vi "LoadOrCreateAParaIniCfg.vi"(8 "error in":errorcluster, 10 "Tree Refnum":refnum<vi>, 11 "Tbl Refnum in":refnum<vi>) -> (0 "error out":errorcluster, 1 "cfg file refnum out":refnum<file>, 2 "Tree Refnum out":refnum<vi>, 3 "Tbl Refnum out":refnum<vi>)   [LabVIEW 2010]
panel:
  out "All Tags":string[](array[string])
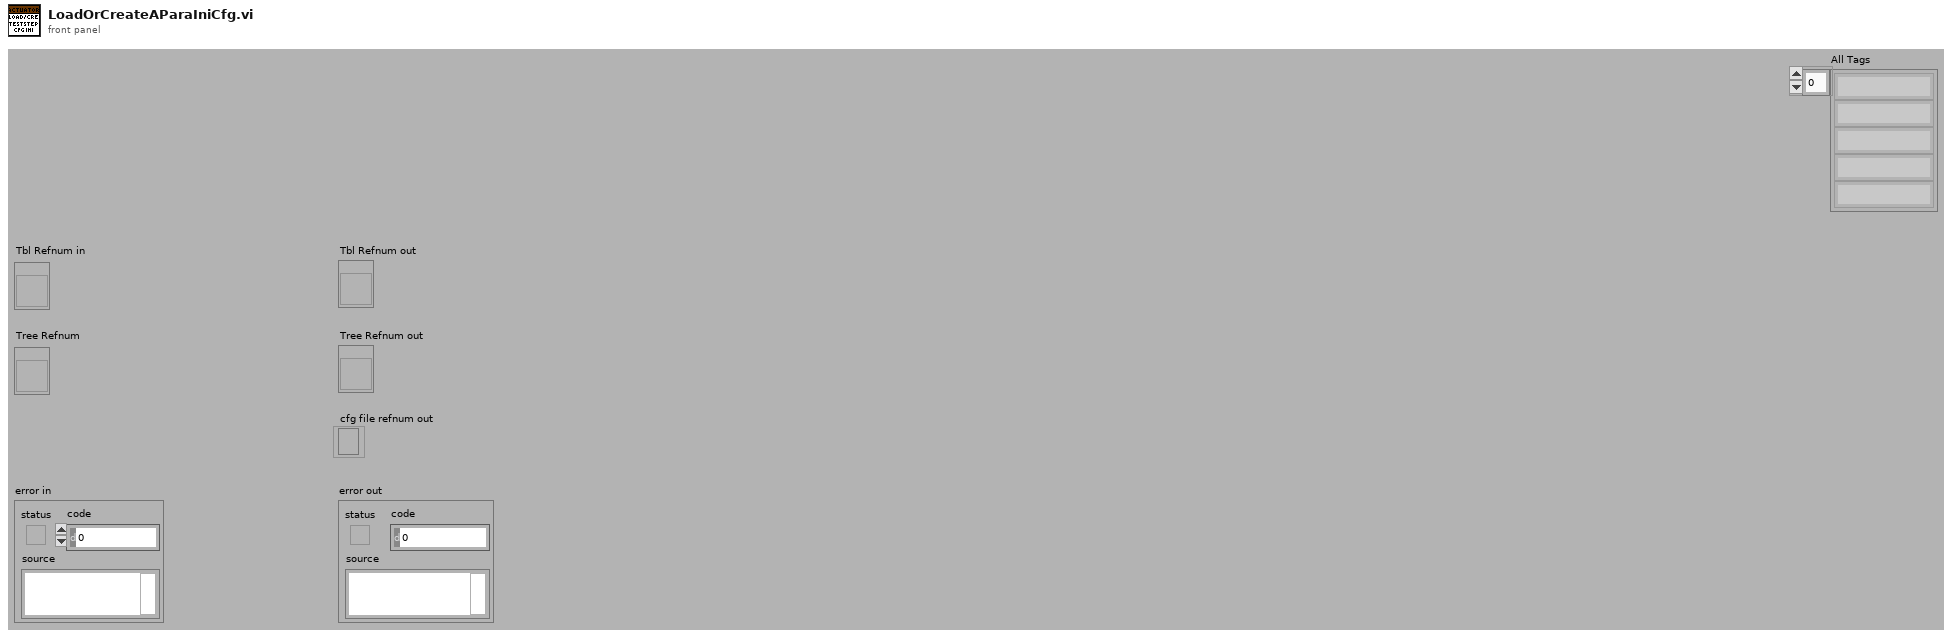
[diagram p1: front panel]
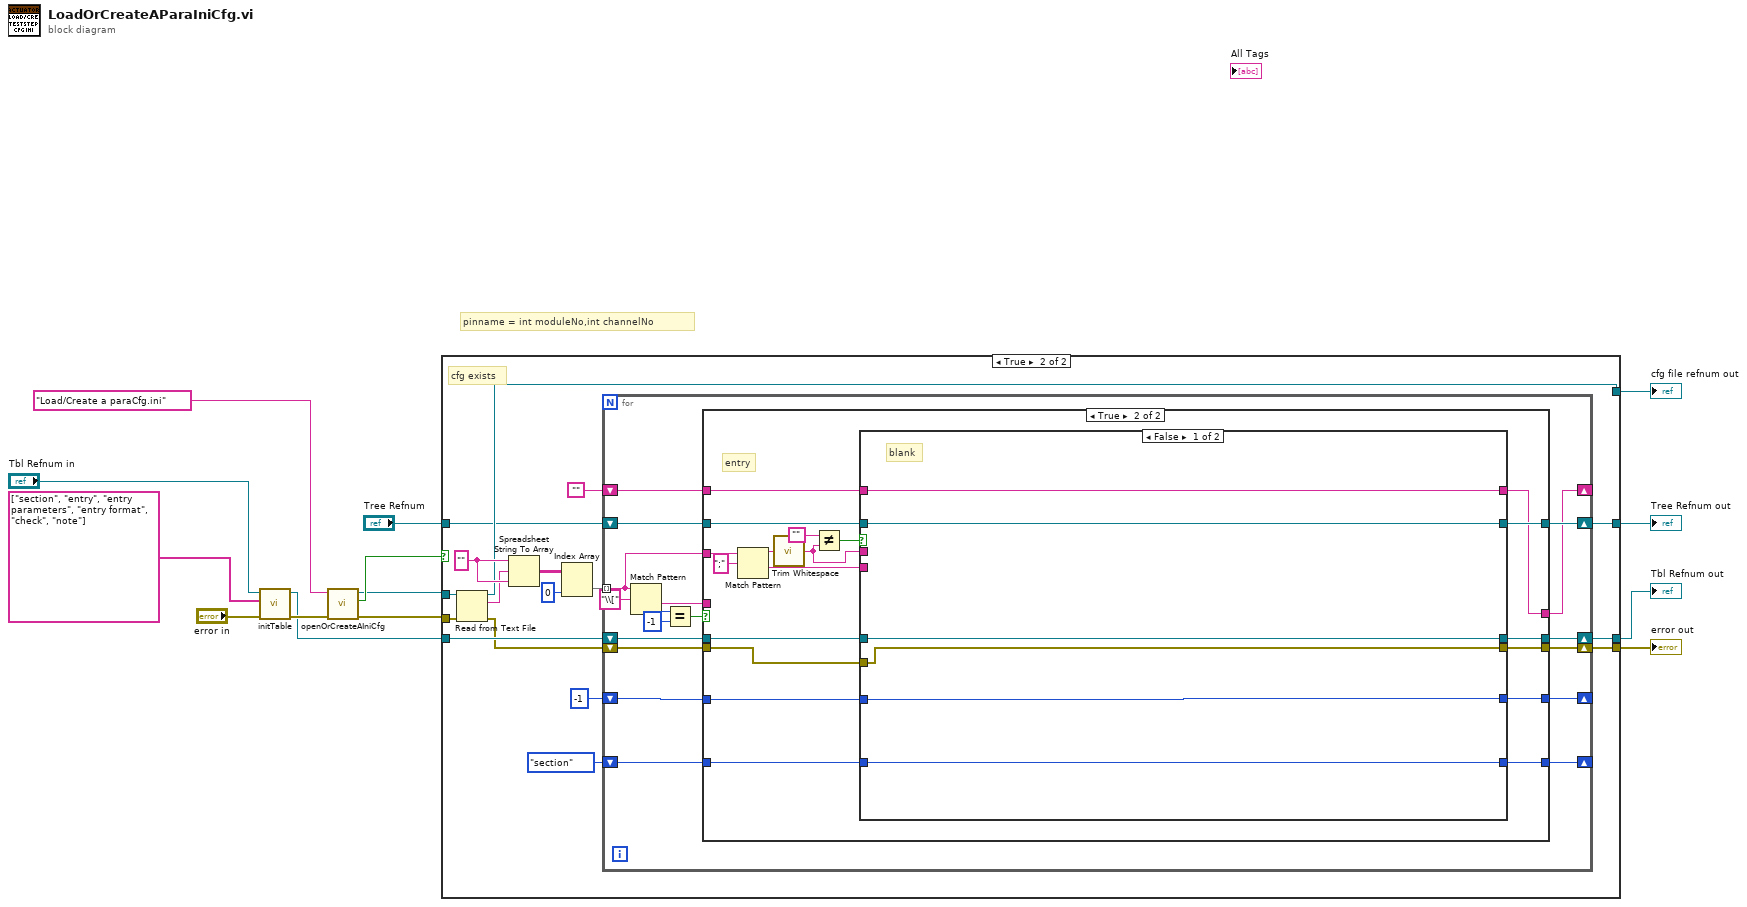
[diagram p0: block diagram]
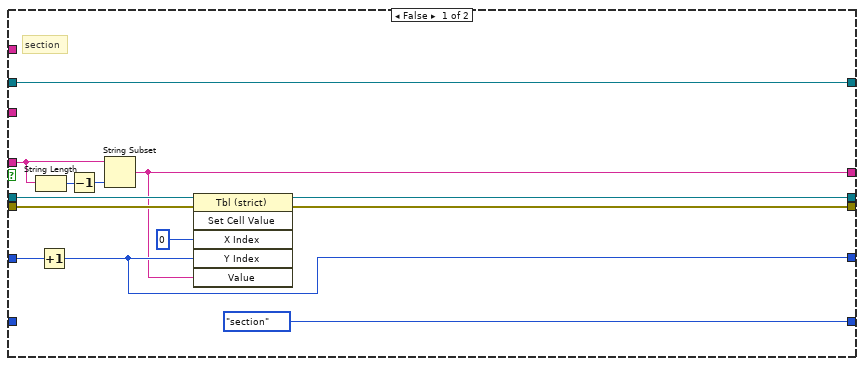
[diagram p3: hidden frame]
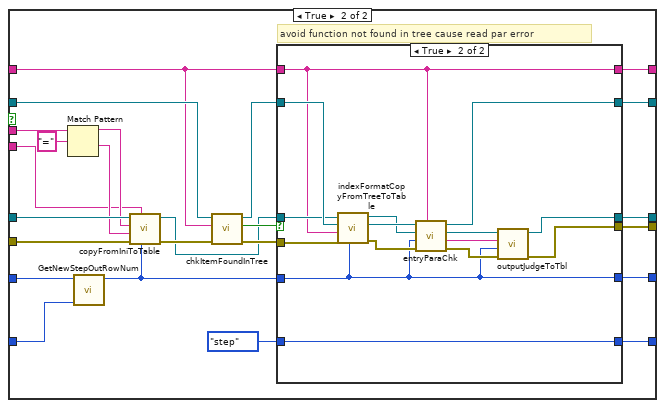
[diagram p4: hidden frame]
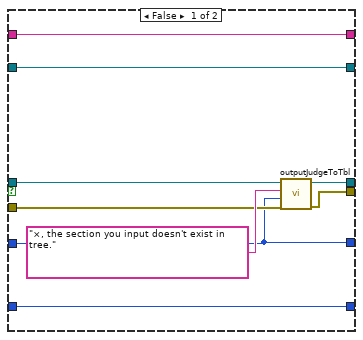
[diagram p5: hidden frame]
diagram:
  # "pinname = int moduleNo,int channelNo"
  n1 = call "initTable.vi"("error in"="error in", "Column Header Strings[]"=string[] ["section", "entry", "entry parameters", "entry format", "check", "note"] ("Row Header Strings[]"), "Tbl Refnum in"="Tbl Refnum in") -> ("error out"=w7:errorcluster, "Tbl Refnum out"=w2:refnum<vi>)  [unwired: 7 in]
  n2 = call "openOrCreateAIniCfg.vi"("error in"=w7, "prompt"="Load/Create a paraCfg.ini") -> ("error out"=w3:errorcluster, "exists"=w5:bool, "ini refnum out"=w4:refnum<file>)  [unwired: 7 in]
  n3 = case shown="True" w5 {
    tunnel: w4 -> [w18 w31]
    tunnel: w3 -> [w17 w30]
    tunnel: w2 -> [w16 w28]
    tunnel: [w18 w25] -> w14
    tunnel: [w17 w24] -> w13
    tunnel: [w16 w22] -> w12
    tunnel: "Tree Refnum" -> [w15 w21]
    tunnel: [w15 w20] -> w10
    frame False {
      # "create a new cfg"
    }
    frame True {
      w33 = ""
      # "cfg exists"
      n4 = Read from Text File(file (use dialog)=w31, error in=w30) -> (refnum out=w25:refnum<file>, text=w32:string, error out=w23:errorcluster)  [unwired: 2 in, 1 out]
      n5 = Spreadsheet String To Array(format string=w33, spreadsheet string=w32, array type (2D Dbl)=w33) -> (array=w34:string[][])  [unwired: 1 in]
      n6 = Index Array(array=w34, index (col)=0 ("disabled index (col)")) -> (element=w29:string[])  [unwired: 1 in]
      n7 = for {
        tunnel: w29 -> [w47] mode=indexing
        shift-right: [w45] -> _
        shift-left: -1 -> [w49]
        shift-right: [w44] -> _
        shift-left: enum16{"section", "step"}."section" -> [w43]
        shift-right: [w42] -> w24
        shift-left: w23 -> [w41]
        shift-right: [w40] -> w22
        shift-left: w28 -> [w46]
        shift-right: [w38] -> w20
        shift-left: w21 -> [w39]
        shift-right: [w37] -> _
        shift-left: "" -> [w36]
        n8 = Match Pattern(string=w47, regular expression="\\[") -> (after substring=w48:string, offset past match=w52:i32)  [unwired: 1 in, 2 out]
        n9 = Equal?(x=w52, y=-1) -> (x = y?=w50:bool)
        n10 = case shown="True" w50 {
          tunnel: w49 -> [w61 w84]
          tunnel: [w60 w83] -> w45
          tunnel: w48 -> [w66 _]
          tunnel: w47 -> [_ w77]
          tunnel: w46 -> [w63 w85]
          tunnel: [enum16{"section", "step"}."section" w82] -> w44
          tunnel: w43 -> [_ w81]
          tunnel: w41 -> [w58 w80]
          tunnel: [w57 w79] -> w42
          tunnel: [w56 w78] -> w40
          tunnel: w39 -> [w55 w73]
          tunnel: [w55 w75] -> w38
          tunnel: [w54 w71] -> w37
          tunnel: w36 -> [_ w72]
          frame False {
            # "section"
            n11 = String Length(string=w66) -> (length=w65:i32)
            n12 = Increment(x=w61) -> (x+1=w60:i32)
            n13 = Decrement(x=w65) -> (x-1=w64:i32)
            n14 = String Subset(string=w66, length (rest)=w64) -> (substring=w54:string)  [unwired: 1 in]
            n15 = invoke class="Tbl (strict)" method="Set Cell Value"(reference=w63, error in=w58, "X Index"=u32 0 ("Y Index"), "Y Index"=w60, "Value"=w54) -> (reference out=w56:refnum<vi>, error out=w57:errorcluster)  [unwired: 1 in, 4 out]
          }
          frame True {
            # "entry"
            n16 = Match Pattern(string=w77, regular expression=";") -> (before substring=w70:string, after substring=w74:string)  [unwired: 1 in, 2 out]
            n17 = call <vilib>:"Trim Whitespace.vi"("string"=w70) -> ("trimmed string"=w67:string)  [unwired: 1 in]
            n18 = Not Equal?(x="", y=w67) -> (x != y?=w68:bool)
            n19 = case shown="False" w68 {
              tunnel: w85 -> [w88 w115]
              tunnel: w84 -> [w91 w114]
              tunnel: [w91 w113] -> w83
              tunnel: [w90 w112] -> w82
              tunnel: w81 -> [w90 w111]
              tunnel: w80 -> [w89 w110]
              tunnel: [w89 w109] -> w79
              tunnel: [w88 w108] -> w78
              tunnel: [w87 w107] -> w75
              tunnel: w74 -> [_ w102]
              tunnel: w73 -> [w87 w101]
              tunnel: w72 -> [w86 w94]
              tunnel: [w86 w93] -> w71
              tunnel: w67 -> [_ w92]
              frame False {
                # "blank"
              }
              frame True {
                # "avoid function not found in tree cause read par error"
                n20 = Match Pattern(string=w92, regular expression="=") -> (before substring=w104:string, after substring=w103:string)  [unwired: 1 in, 2 out]
                n21 = call "GetNewStepOutRowNum.vi"("lastStat"=w111, "lastRowNum"=w114) -> ("outRowNum"=w98:i32)  [unwired: 9 in]
                n22 = call "copyFromIniToTable.vi"("tableRowNum"=w98, "valInCol5"=w102, "error in"=w110, "valInCol2"=w103, "valInCol1"=w104, "Tbl Refnum in"=w115) -> ("error out"=w100:errorcluster, "Tbl Refnum out"=w95:refnum<vi>)  [unwired: 4 in]
                n23 = call "chkItemFoundInTree.vi"("error in"=w100, "searchItem"=w94, "Tree Refnum in"=w101) -> ("error out"=w99:errorcluster, "FoundInTree?"=w97:bool, "Tree Refnum out"=w96:refnum<vi>)  [unwired: 6 in]
                n24 = case shown="True" w97 {
                  tunnel: [w124 w138] -> w107
                  tunnel: w96 -> [w124 w137]
                  tunnel: [w120 w129] -> w108
                  tunnel: [w119 w128] -> w109
                  tunnel: w98 -> [w118 w131]
                  tunnel: enum16{"section", "step"}."step" -> [w117 w139]
                  tunnel: [w117 w139] -> w112
                  tunnel: [w118 w131] -> w113
                  tunnel: w95 -> [w123 w127]
                  tunnel: w99 -> [w121 w126]
                  tunnel: w94 -> [w116 w125]
                  tunnel: [w116 w125] -> w93
                  frame False {
                    n25 = call "outputJudgeToTbl.vi"("error in"=w121, "rowNum"=w118, "judgeRes"="×, the section you input doesn't exist in tree." ("Value"), "Tbl Refnum in"=w123) -> ("error out"=w119:errorcluster, "Tbl Refnum Out"=w120:refnum<vi>)  [unwired: 6 in]
                  }
                  frame True {
                    n26 = call "indexFormatCopyFromTreeToTable.vi"("rowNum"=w131, "error in"=w126, "searchItem"=w125, "Tree Refnum In"=w137, "Tbl Refnum in"=w127) -> ("error out"=w134:errorcluster, "Tree Refnum Out"=w136:refnum<vi>, "Tbl Refnum Out"=w135:refnum<vi>)  [unwired: 4 in]
                    n27 = call "entryParaChk.vi"("indexSec"=w125, "error in"=w134, "Row number"=w131, "Tbl Refnum in"=w135, "Tree Refnum in"=w136) -> ("error out"=w132:errorcluster, "Check result"=w130:string, "Tbl Refnum out"=w133:refnum<vi>, "Tree Refnum out"=w138:refnum<vi>)  [unwired: 3 in]
                    n28 = call "outputJudgeToTbl.vi"("error in"=w132, "rowNum"=w131, "judgeRes"=w130, "Tbl Refnum in"=w133) -> ("error out"=w128:errorcluster, "Tbl Refnum Out"=w129:refnum<vi>)  [unwired: 6 in]
                  }
                }
              }
            }
          }
        }
      }
    }
  }
  "error out" <- w13
  "cfg file refnum out" <- w14
  "Tbl Refnum out" <- w12
  "Tree Refnum out" <- w10
